vi "Apply Video Prefs.vi"(8 "error in (no error)":errorcluster, 10 "Video Prefs":T1, 11 "SB App in":refnum<class "SB App.lvclass">) -> (0 "error out":errorcluster, 3 "SB App out":refnum<class "SB App.lvclass">)   [LabVIEW 2020, in "SB App.lvlib" / "SB App.lvclass"]
uses:
  SB App.lvclass
  SB App.lvclass/SB App.ctl
  df9730b3-62a7-4eac-8a00-b176b9cff08e.vi
  05510a1c-28c7-49ff-b3f4-2f5932124493.vi
  Video Prefs.ctl
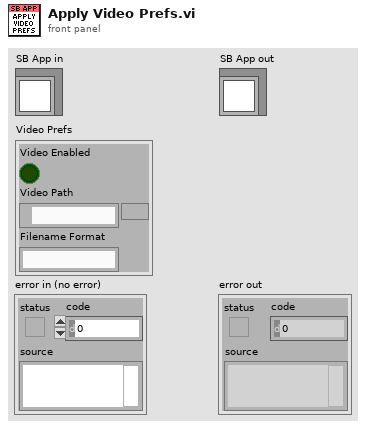
[diagram p1: front panel]
types:
  T1 = typedef "SB App.lvlib/SB App.lvclass/Video Prefs.ctl" = cluster{"Video Enabled":bool, "Video Path":path, "Filename Format":string}
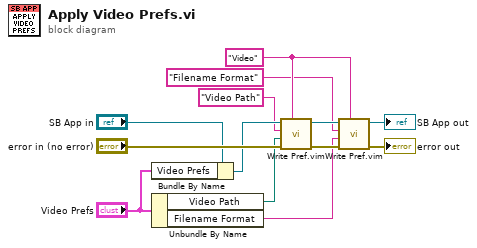
[diagram p0: block diagram]
diagram:
  w5 = "Video" ("Section")
  n1 = Bundle By Name(cluster="SB App in", "Video Prefs"="Video Prefs") -> (w9:refnum<class "SB App.lvclass">)
  n2 = Unbundle By Name("Video Prefs") -> ("Video Path"=w7:path, "Filename Format"=w3:string)
  n3 = call "Write Pref.vim"("Section"=w5, "error in (no error)"="error in (no error)", "Value"=w7, "Key"="Video Path", "SB App in"=w9) -> ("error out"=w13:errorcluster, "SB App out"=w6:refnum<class "SB App.lvclass">)  [unwired: 5 in]
  n4 = call "Write Pref.vim"("Section"=w5, "error in (no error)"=w13, "Value"=w3, "Key"="Filename Format", "SB App in"=w6) -> ("error out"=→"error out":errorcluster, "SB App out"=→"SB App out":refnum<class "SB App.lvclass">)  [unwired: 5 in]
